vi "write_9264_output.vi"(6 "Channel":T1={"Operation"=0, "Num. Steps"=0, "Begin"=0.0, "Step Size"=0.0, "Input - A"=0, "Input - B"=0, "Output - LO"=0.0, "Output - HI"=0.0, "Reset"=FALSE, "Analog Output"=0, "Trigger Input"=0, "Initialize To"=0, "Digital Inputs"=[0, 0, 0, 0, 0], "Output Values"=[0.0, 0.0, 0.0, 0.0, 0.0], "Num. Inputs"=4} {"Digital Inputs" items=["DIO0", "DIO1", "DIO2", "DIO3", "DIO4", "DIO5", "DIO6", "DIO7", "DIO8", "DIO9", "DIO10", "DIO11", "DIO12", "DIO13", "DIO14", "DIO15", "DIO16", "DIO17", "DIO18", "DIO19", "DIO20", "DIO21", "DIO22", "DIO23", "DIO24", "DIO25", "DIO26", "DIO27", "DIO28", "DIO29", "DIO30", "DIO31"]; "Initialize To" items=["Zero", "Begin Value"]; "Trigger Input" items=["DIO0", "DIO1", "DIO2", "DIO3", "DIO4", "DIO5", "DIO6", "DIO7", "DIO8", "DIO9", "DIO10", "DIO11", "DIO12", "DIO13", "DIO14", "DIO15", "DIO16", "DIO17", "DIO18", "DIO19", "DIO20", "DIO21", "DIO22", "DIO23", "DIO24", "DIO25", "DIO26", "DIO27", "DIO28", "DIO29", "DIO30", "DIO31"]; "Analog Output" items=["AO\\00", "AO\\01", "AO\\02", "AO\\03", "AO\\04", "AO\\05", "AO\\06", "AO\\07", "AO\\08", "AO\\09", "AO\\10", "AO\\11", "AO\\12", "AO\\13", "AO\\14", "AO\\15"]; "Input - B" items=["DIO0", "DIO1", "DIO2", "DIO3", "DIO4", "DIO5", "DIO6", "DIO7", "DIO8", "DIO9", "DIO10", "DIO11", "DIO12", "DIO13", "DIO14", "DIO15", "DIO16", "DIO17", "DIO18", "DIO19", "DIO20", "DIO21", "DIO22", "DIO23", "DIO24", "DIO25", "DIO26", "DIO27", "DIO28", "DIO29", "DIO30", "DIO31"]; "Input - A" items=["DIO0", "DIO1", "DIO2", "DIO3", "DIO4", "DIO5", "DIO6", "DIO7", "DIO8", "DIO9", "DIO10", "DIO11", "DIO12", "DIO13", "DIO14", "DIO15", "DIO16", "DIO17", "DIO18", "DIO19", "DIO20", "DIO21", "DIO22", "DIO23", "DIO24", "DIO25", "DIO26", "DIO27", "DIO28", "DIO29", "DIO30", "DIO31"]; "Operation" items=["OFF", "SWITCH", "AND GATE", "OR GATE", "ITERATION", "CUSTOM - 461nm Freq."]}, 9 "AO Values":fxp<+/-,20,5>[](array[numeric])=[0.0, 0.0, 0.0, 0.0, 0.0, 0.0, 0.0, 0.0, 0.0, 0.0, 0.0, 0.0, 0.0, 0.0, 0.0, 0.0]) -> ()   [LabVIEW 2016]
uses:
  fpga_array_element.ctl
  <vilib>/rvi/eio/common/nirviEmuTemplateMethod_errors.vi
  <vilib>/eio/EIONode/EIONode.xnode
panel:
  # "Boolean Operation Controls"
  # "Iteration Operation Controls"
  # "Custom Operation Controls"
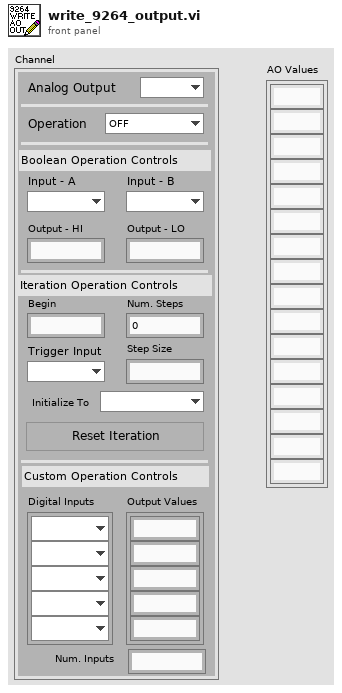
[diagram p1: front panel]
types:
  T1 = typedef "fpga_array_element.ctl" = cluster{"Operation":i16, "Num. Steps":u16, "Begin":fxp<+/-,20,5>, "Step Size":fxp<+/-,20,5>, "Input - A":i32, "Input - B":i32, "Output - LO":fxp<+/-,20,5>, "Output - HI":fxp<+/-,20,5>, "Reset":bool, "Analog Output":i32, "Trigger Input":i32, "Initialize To":i16, "Digital Inputs":i32[], "Output Values":fxp<+/-,20,5>[], "Num. Inputs":u16}
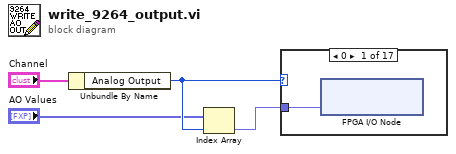
[diagram p0: block diagram]
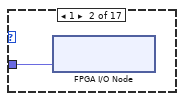
[diagram p2: hidden frame]
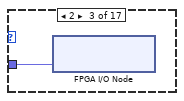
[diagram p3: hidden frame]
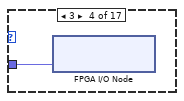
[diagram p4: hidden frame]
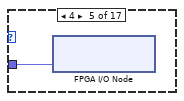
[diagram p5: hidden frame]
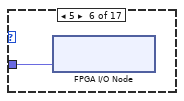
[diagram p6: hidden frame]
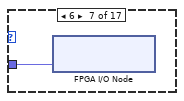
[diagram p7: hidden frame]
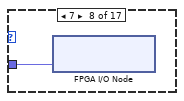
[diagram p8: hidden frame]
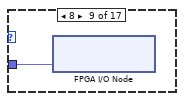
[diagram p9: hidden frame]
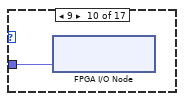
[diagram p10: hidden frame]
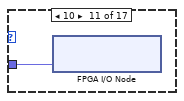
[diagram p11: hidden frame]
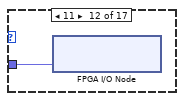
[diagram p12: hidden frame]
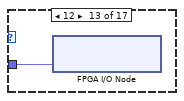
[diagram p13: hidden frame]
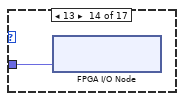
[diagram p14: hidden frame]
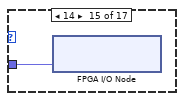
[diagram p15: hidden frame]
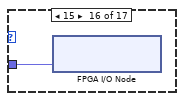
[diagram p16: hidden frame]
diagram:
  n1 = Unbundle By Name("Channel") -> ("Analog Output"=w3:i32)
  n2 = Index Array(array="AO Values", index=w3) -> (element=w1:fxp<+/-,20,5>)
  n3 = case shown="0" w3 {
    tunnel: w1 -> [w5 w6 w7 w8 w9 w10 w11 w12 w13 w14 w15 w16 w17 w18 w19 w20 _]
    frame 0 {
      n4 = xnode "FPGA I/O Node"("Mod4/AO0"=w5) -> ()  [unwired: 1 in, 1 out]
    }
    frame 1 {
      n5 = xnode "FPGA I/O Node"("Mod4/AO1"=w6) -> ()  [unwired: 1 in, 1 out]
    }
    frame 2 {
      n6 = xnode "FPGA I/O Node"("Mod4/AO2"=w7) -> ()  [unwired: 1 in, 1 out]
    }
    frame 3 {
      n7 = xnode "FPGA I/O Node"("Mod4/AO3"=w8) -> ()  [unwired: 1 in, 1 out]
    }
    frame 4 {
      n8 = xnode "FPGA I/O Node"("Mod4/AO4"=w9) -> ()  [unwired: 1 in, 1 out]
    }
    frame 5 {
      n9 = xnode "FPGA I/O Node"("Mod4/AO5"=w10) -> ()  [unwired: 1 in, 1 out]
    }
    frame 6 {
      n10 = xnode "FPGA I/O Node"("Mod4/AO6"=w11) -> ()  [unwired: 1 in, 1 out]
    }
    frame 7 {
      n11 = xnode "FPGA I/O Node"("Mod4/AO7"=w12) -> ()  [unwired: 1 in, 1 out]
    }
    frame 8 {
      n12 = xnode "FPGA I/O Node"("Mod4/AO8"=w13) -> ()  [unwired: 1 in, 1 out]
    }
    frame 9 {
      n13 = xnode "FPGA I/O Node"("Mod4/AO9"=w14) -> ()  [unwired: 1 in, 1 out]
    }
    frame 10 {
      n14 = xnode "FPGA I/O Node"("Mod4/AO10"=w15) -> ()  [unwired: 1 in, 1 out]
    }
    frame 11 {
      n15 = xnode "FPGA I/O Node"("Mod4/AO11"=w16) -> ()  [unwired: 1 in, 1 out]
    }
    frame 12 {
      n16 = xnode "FPGA I/O Node"("Mod4/AO12"=w17) -> ()  [unwired: 1 in, 1 out]
    }
    frame 13 {
      n17 = xnode "FPGA I/O Node"("Mod4/AO13"=w18) -> ()  [unwired: 1 in, 1 out]
    }
    frame 14 {
      n18 = xnode "FPGA I/O Node"("Mod4/AO14"=w19) -> ()  [unwired: 1 in, 1 out]
    }
    frame 15 {
      n19 = xnode "FPGA I/O Node"("Mod4/AO15"=w20) -> ()  [unwired: 1 in, 1 out]
    }
    frame 16, Default {
    }
  }
